vi "my IP addresses.vi"() -> (0 "number of addresses":i32, 3 "available IP addresses":string[](array[string]))   [LabVIEW 2017]
panel:
  # "my IP addresses"
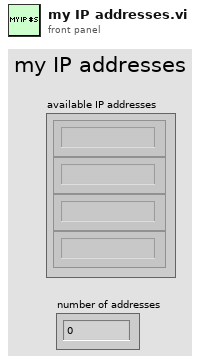
[diagram p1: front panel]
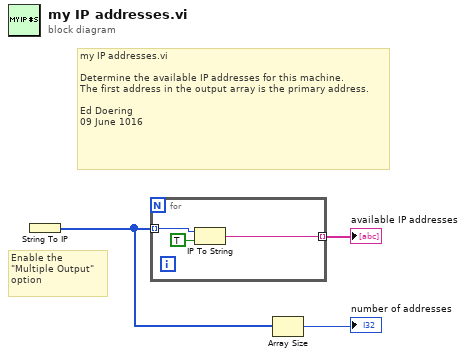
[diagram p0: block diagram]
diagram:
  # "Enable the\n\"Multiple Output\"\noption"
  # "my IP addresses.vi\n\nDetermine the available IP addresses for this machine.\nThe first address in the output array is the primary address.\n\nEd Doering\n09 June 1016"
  n1 = String To IP() -> (0:w2:u32[])  [unwired: 1 in]
  n2 = for {
    tunnel: w2 -> [w5] mode=indexing
    tunnel: [w4] -> w3 mode=indexing
    n3 = IP To String(1:TRUE ("dot notation? (F)"), 2:w5) -> (0:w4:string)
  }
  "available IP addresses" <- w3
  n4 = Array Size(array=w2) -> (size(s)=→"number of addresses":i32)
